vi "scan nufern reply string.vi"(0 "Input String":string, 2 "Manual":bool, 5 "error in (no error)":errorcluster={"status"=FALSE, "code"=0, "source"="No Error."}) -> (6 "Laser is in High Power Mode":bool, 8 "Status Cluster":T2, 9 "HPE Photodiode Reading":u32 format="0x%08x", 10 "Fault Cluster":T1, 11 "Back-Reflection Reading":u32 format="0x%08x", 13 "Return Code Cluster":T7 {"Current RS-485 \nAddress" format="0x%02x"; "Desired RS-485 \nAddress" format="0x%02x"; "Set Power Mode Return Code" format="0x%02x"; "Clear Faults Return Code" format="0x%02x"; "Return Code Description" items=["Accepted/No Error", "Incorrect Message Format", "Incorrect Message Length", "CRC Error", "Unrecognized Command", "Argument Out of Range", "Argument Parse Error", "Operation Not Permitted", "Operation Failed"]; "Get RS-485 Address \nReturn Code" format="0x%02x"; "Set RS-485 Address \nReturn Code" format="0x%02x"; "Set Power Mode Return Code" format="0x%02x"; "Clear Faults Return Code" format="0x%02x"; "Extended Status Return Code" format="0x%02x"}, 14 "New value is outside \nof the inclusive range of 1-99%":bool, 15 "New Value Could not be parsed":bool, 16 "Fault Status Cluster":T5, 17 "Extended Status Cluster":T4 {"Temperature Array" format="0x%02x"; "Back-Reflection" format="0x%08x"; "HPE Threshold" format="0x%08x"; "HPE Monitor" format="0x%08x"; "Stage 2 Output Monitor" format="0x%08x"; "Stage 1 Input Monitor" format="0x%08x"; "Stage 2 Current" format="0x%08x"; "Stage 1 Current" format="0x%08x"; "Extended Status Return Code" format="0x%02x"}, 18 "Unit Status Cluster":T6={"laser serial number"=0, "Firmware Part Number"=0, "Firmware Version Major"=1, "Firmware Version Minor"=1, "Firmware Version Bugfix"=1, "Gateware Part Number"=0, "Gateware Version Minor"=1, "Gateware Version Major"=1, "Gateware Version Bugfix"=1, "Valid Readings"=FALSE} {"Gateware Version Bugfix" format="0x%02x"; "Gateware Version Major" format="0x%02x"; "Gateware Version Minor" format="0x%02x"; "Gateware Part Number" format="0x%04x"; "Firmware Version Bugfix" format="0x%02x"; "Firmware Version Minor" format="0x%02x"; "Firmware Version Major" format="0x%02x"; "Firmware Part Number" format="0x%04x"}, 19 "error out":errorcluster)   [LabVIEW 2016]
uses:
  sniper current tests/Return Code Cluster.ctl
  2 digit hex indicator.ctl
  sniper current tests/Unit Status Cluster Control 1.ctl
  sniper current tests/Status  Cluster.ctl
  sniper current tests/Fault Cluster.ctl
panel:
  out "Logistics":u16(ring)=65 items=["Set RS-485 Address"=65, "Get RS-485 Address"=66]
  out "Common Operation":u16(ring) items=["undetermined", "Get Unit Information", "Emission On", "Emission Off", "Get Basic Status", "Get Core Status", "Get Extended Status", "Clear Faults", "Set Power Mode", ""]
  out "remaining string":string
  out "return code":u32 format="0x%02x"
  in  "String":string
  out "hexadecimal string out":string
  out "CRC Out":i32 format="0x%x"
  out "CRC Valid":bool
  out "Calculated CRC":i32 format="0x%x"
  out "Response string":string
  out "Address  String Out":string
  out "ID word":u32 format="0x%02x"
  out "Address Integer":u32 format="0x%02x"
  out "after address":string
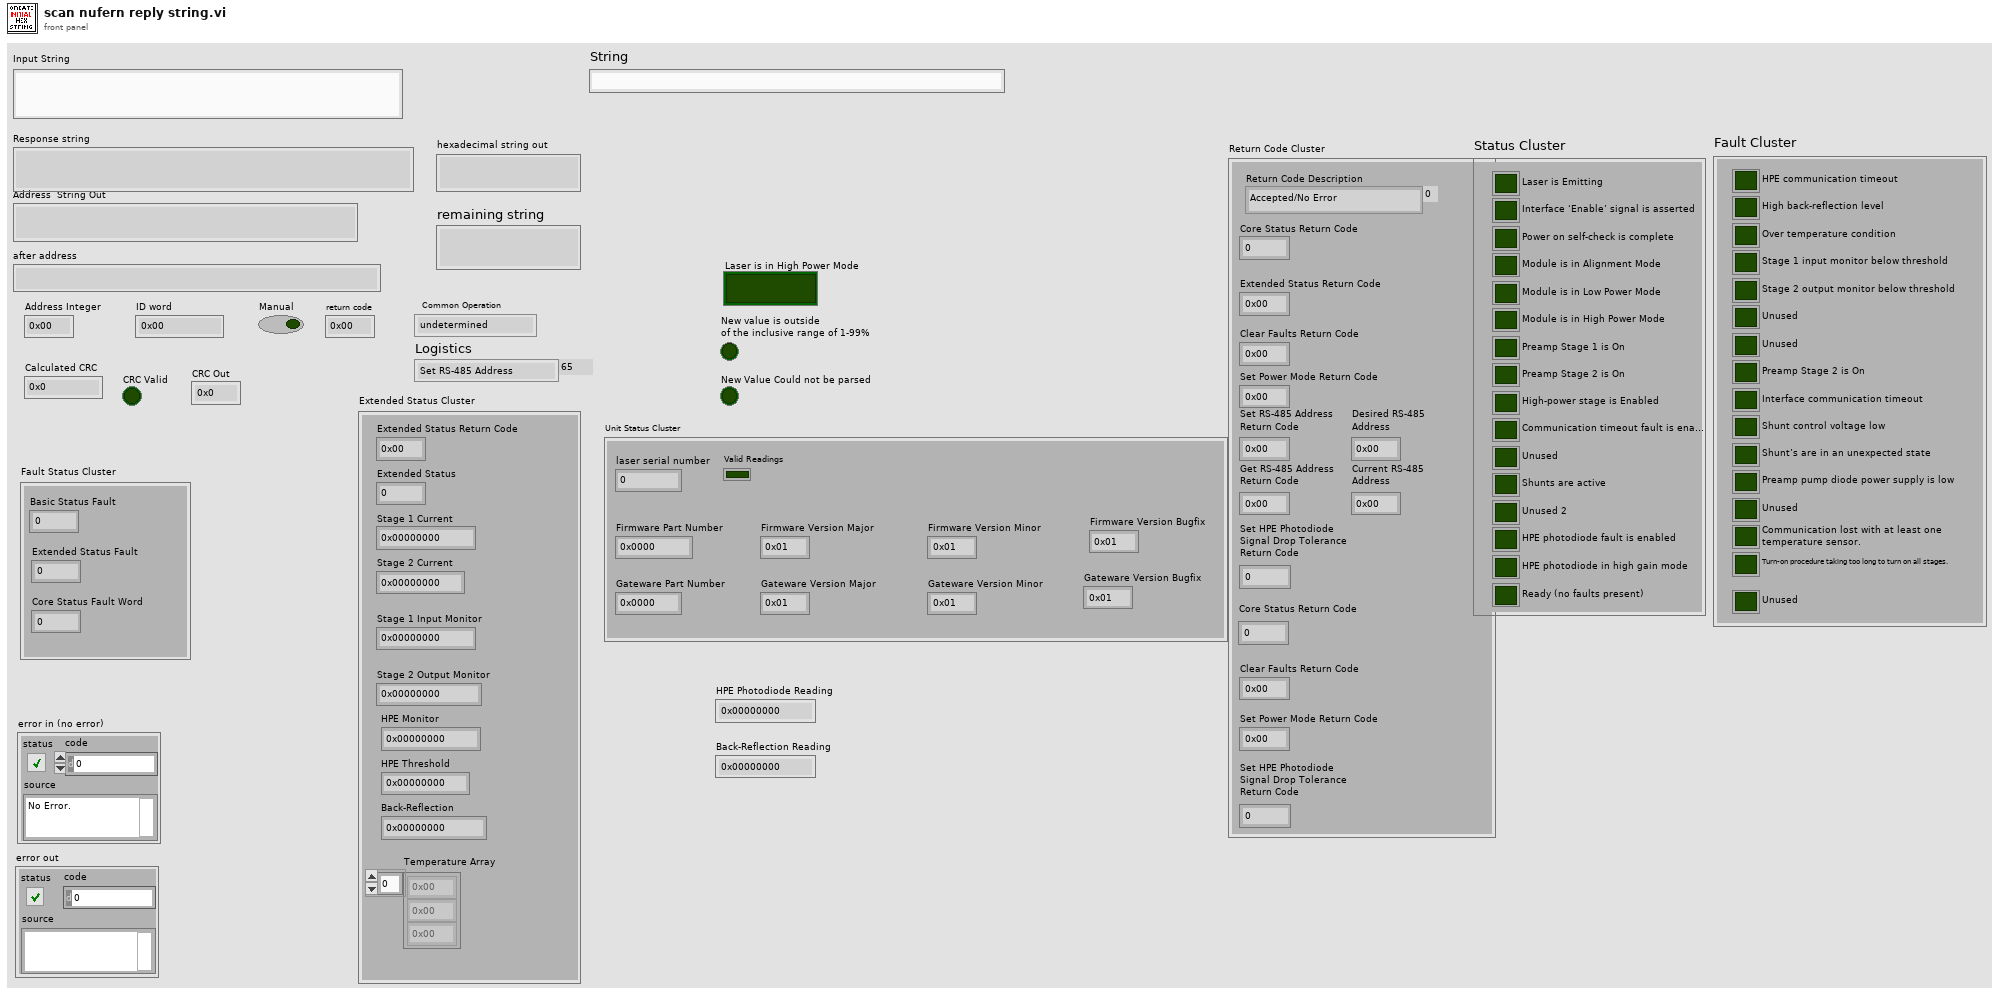
[diagram p1: front panel]
types:
  T1 = typedef "Fault Cluster.ctl" = cluster{"HPE communication timeout":bool, "High back-reflection level":bool, "Over temperature condition":bool, "Stage 1 input monitor below threshold":bool, "Stage 2 output monitor below threshold":bool, "Unused":bool, "Unused":bool, "Preamp Stage 2 is On":bool, "Interface communication timeout":bool, "Shunt control voltage low":bool, "Shunt’s are in an unexpected state":bool, "Preamp pump diode power supply is low":bool, "Unused":bool, "Communication lost with at least one\ntemperature sensor.":bool, "Turn-on procedure taking too long to turn on all stages.":bool, "Unused":bool}
  T2 = typedef "Status  Cluster.ctl" = cluster{"Laser is Emitting":bool, "Interface ‘Enable’ signal is asserted":bool, "Power on self-check is complete":bool, "Module is in Alignment Mode":bool, "Module is in Low Power Mode":bool, "Module is in High Power Mode":bool, "Preamp Stage 1 is On":bool, "Preamp Stage 2 is On":bool, "High-power stage is Enabled":bool, "Communication timeout fault is enabled":bool, "Unused":bool, "Shunts are active":bool, "Unused 2":bool, "HPE photodiode fault is enabled":bool, "HPE photodiode in high gain mode":bool, "Ready (no faults present)":bool}
  T3 = typedef "2 digit hex indicator.ctl" = i32
  T4 = cluster{"Extended Status Return Code":T3, "Extended Status ":u32, "Stage 1 Current":u32, "Stage 2 Current":u32, "Stage 1 Input Monitor":u32, "Stage 2 Output Monitor":u32, "HPE Monitor":u32, "HPE Threshold":u32, "Back-Reflection":u32, "Temperature Array":T3[]}
  T5 = cluster{"Basic Status Fault":u32, "Core Status Fault Word":u32, "Extended Status Fault":u32}
  T6 = typedef "Unit Status Cluster Control 1.ctl" = cluster{"laser serial number":u32, "Firmware Part Number":u32, "Firmware Version Major":T3, "Firmware Version Minor":T3, "Firmware Version Bugfix":T3, "Gateware Part Number":u32, "Gateware Version Minor":T3, "Gateware Version Major":T3, "Gateware Version Bugfix":T3, "Valid Readings":bool}
  T7 = typedef "Return Code Cluster.ctl" = cluster{"Core Status Return Code":u32, "Extended Status Return Code":T3, "Clear Faults Return Code":T3, "Set Power Mode Return Code":T3, "Set RS-485 Address \nReturn Code":T3, "Get RS-485 Address \nReturn Code":T3, "Set HPE Photodiode \nSignal Drop Tolerance \nReturn Code":u32, "Return Code Description":u16, "Core Status Return Code":u32, "Clear Faults Return Code":T3, "Set Power Mode Return Code ":T3, "Desired RS-485 \nAddress ":T3, "Current RS-485 \nAddress ":T3, "Set HPE Photodiode \nSignal Drop Tolerance \nReturn Code ":u32}
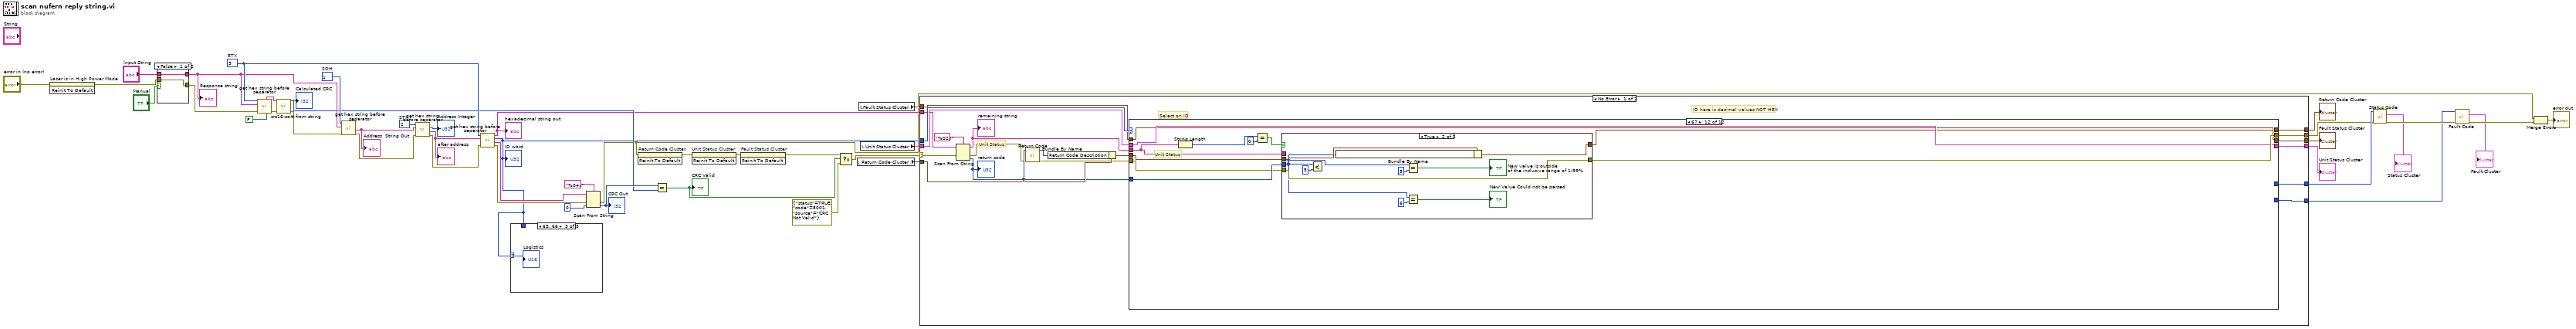
[diagram p0: block diagram]
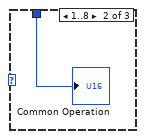
[diagram p3: hidden frame]
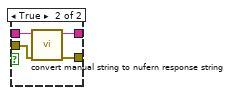
[diagram p4: hidden frame]
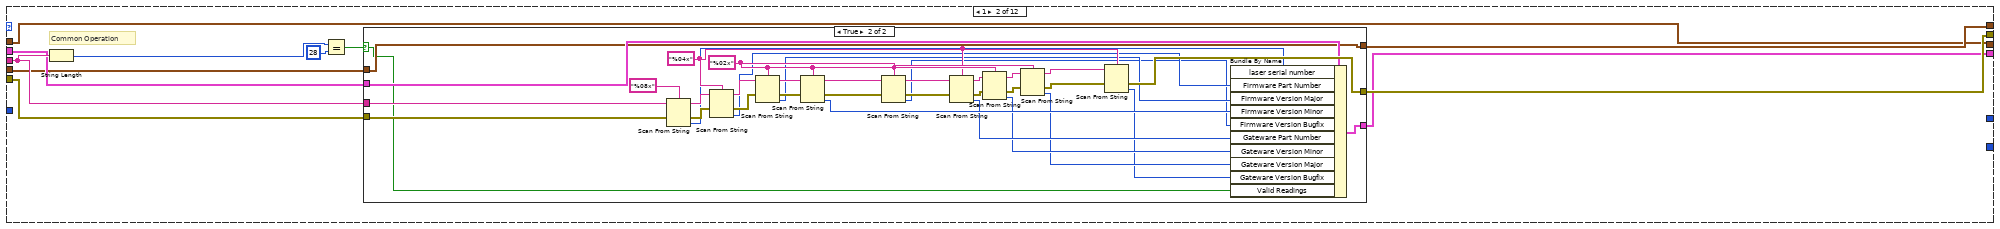
[diagram p6: hidden frame]
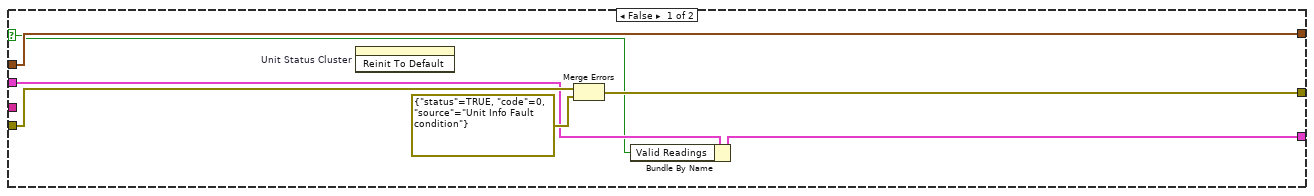
[diagram p7: hidden frame]
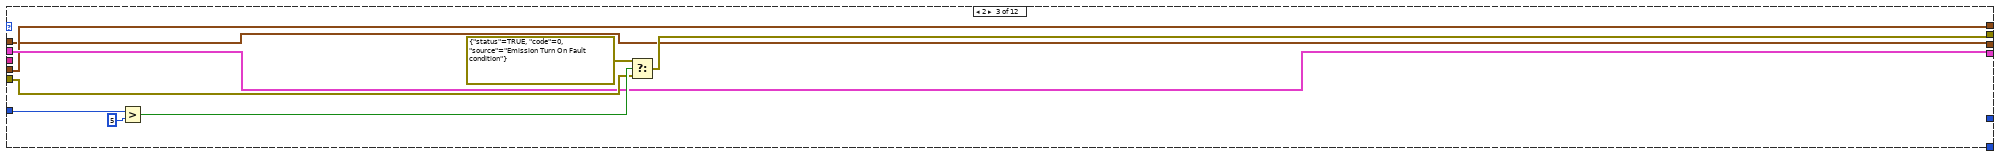
[diagram p8: hidden frame]
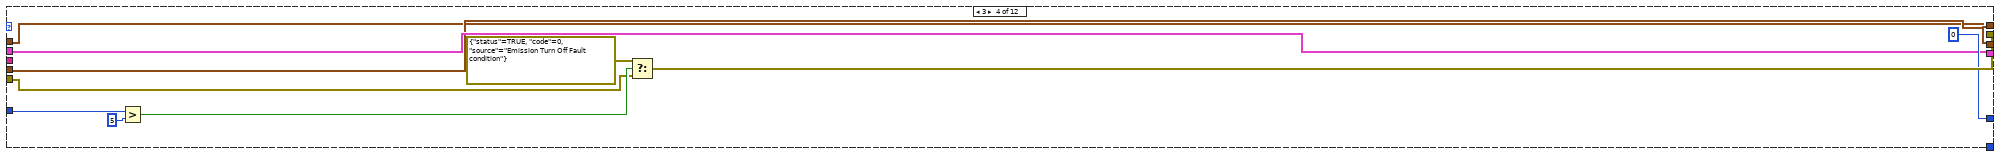
[diagram p9: hidden frame]
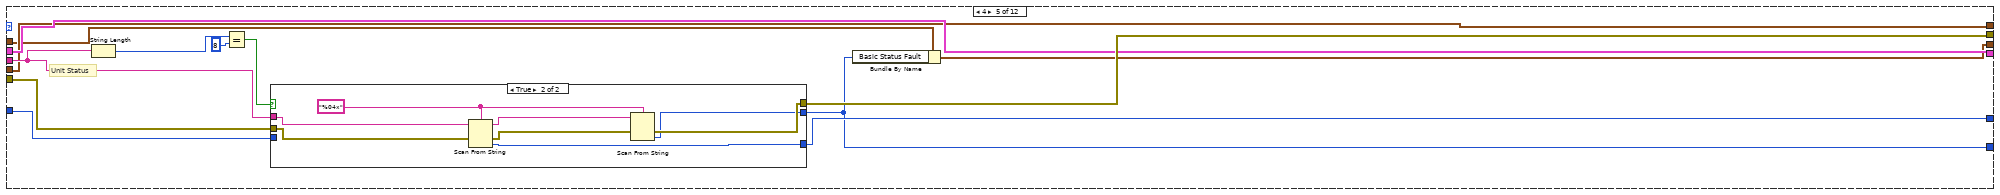
[diagram p10: hidden frame]
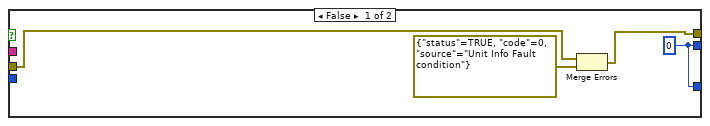
[diagram p11: hidden frame]
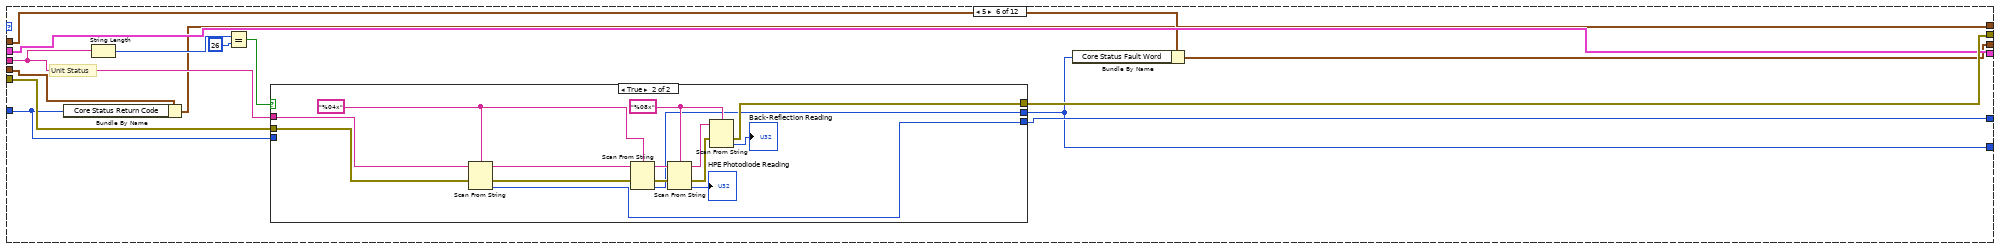
[diagram p12: hidden frame]
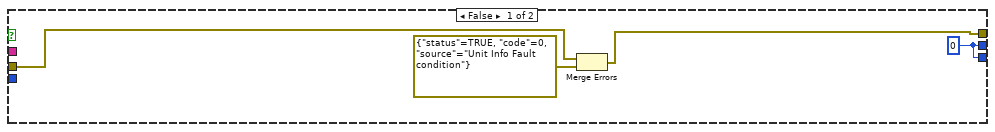
[diagram p13: hidden frame]
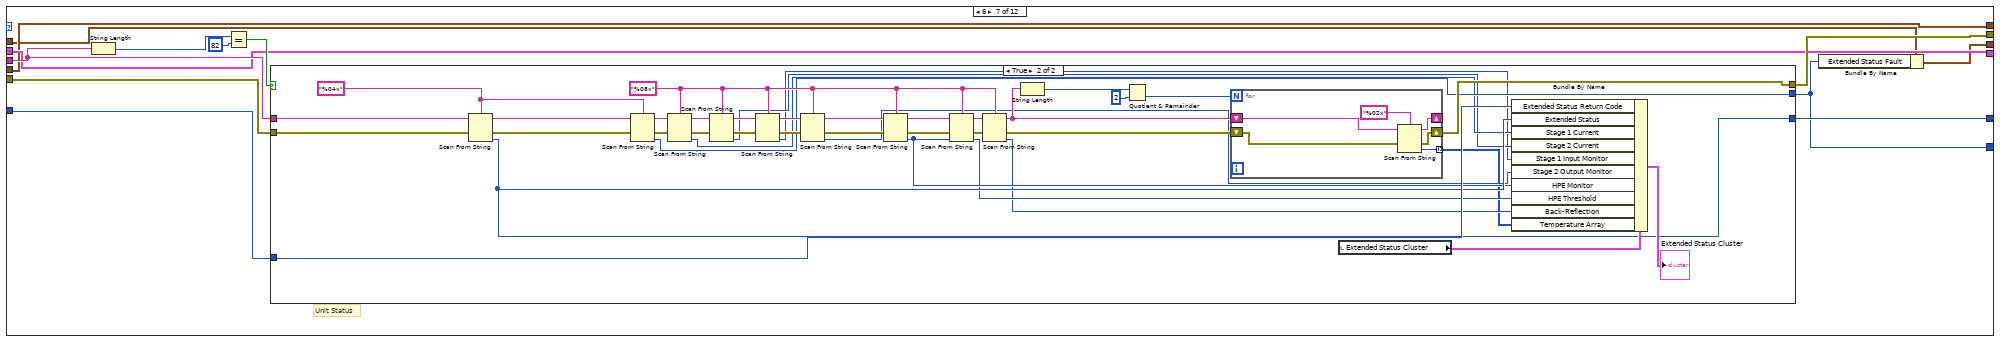
[diagram p14: hidden frame]
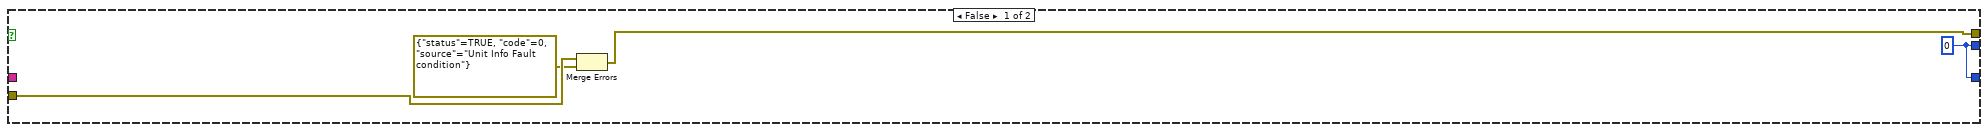
[diagram p15: hidden frame]
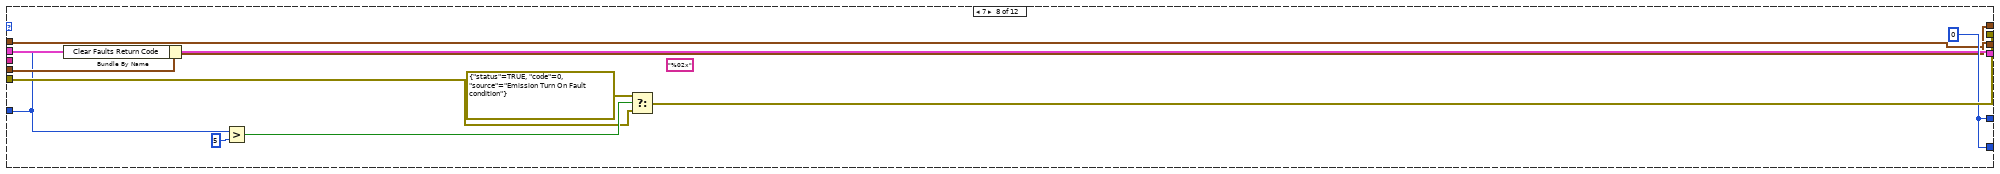
[diagram p16: hidden frame]
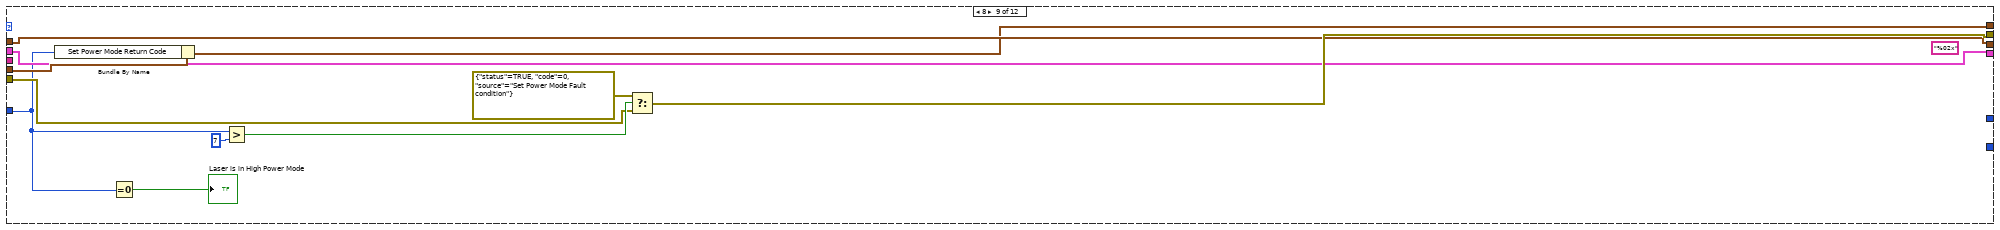
[diagram p17: hidden frame]
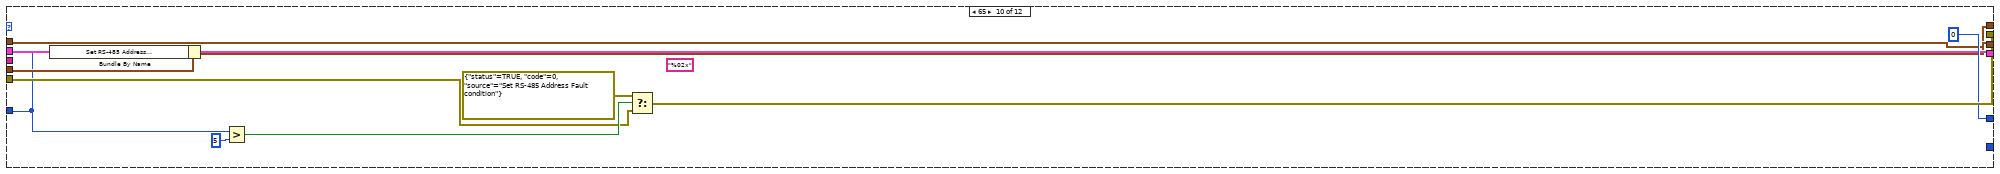
[diagram p18: hidden frame]
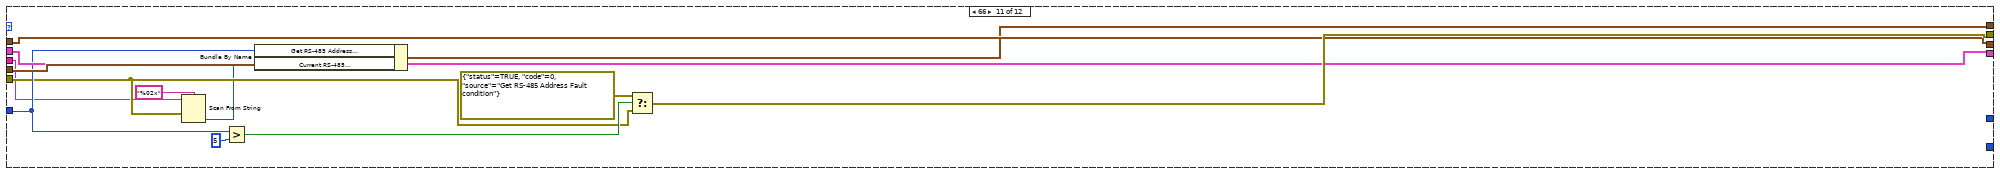
[diagram p19: hidden frame]
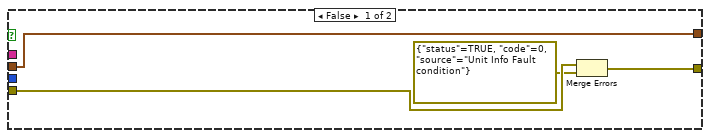
[diagram p20: hidden frame]
diagram:
  w41 = 3  # ETX
  w47 = 2  # STX
  w45 = 1  # SOH
  n1 = invoke on="Laser is in High Power Mode" class="Bool (strict)" method="Reinit To Default"(error in="error in (no error)") -> (error out=w11:errorcluster)  [unwired: 2 in, 2 out]
  n2 = case shown="False" "Manual" {
    tunnel: "Input String" -> [w48 w53]
    tunnel: w11 -> [w49 w52]
    tunnel: [w49 w51] -> w40
    tunnel: [w48 w50] -> w39
    frame False {
    }
    frame True {
      n3 = call "convert manual string to nufern response string.vi"("error in (no error)"=w52, "Manual String"=w53) -> ("error out"=w51:errorcluster, "result string"=w50:string)  [unwired: 8 in]
    }
  }
  "Response string" <- w39
  n4 = call "get hex string before separator.vi"("Convert to hex?"=FALSE, "error in (no error)"=w40, "String In"=w39, "Separator In"=w41) -> ("error out"=w38:errorcluster, "String Before and Separator"=w37:string)  [unwired: 3 in, 3 out]
  n5 = call "crc16-ccitt from string.vi"("error in (no error)"=w38, "String"=w37) -> ("error out"=w36:errorcluster, "CRC Out"=w29:i32)  [unwired: 8 in]
  "Calculated CRC" <- w29
  n6 = call "get hex string before separator.vi"("error in (no error)"=w36, "String In"=w39, "Separator In"=w45) -> ("error out"=w44:errorcluster, "after match out"=w43:string)  [unwired: 4 in, 3 out]
  "Address  String Out" <- w43
  n7 = call "get hex string before separator.vi"("error in (no error)"=w44, "String In"=w43, "Separator In"=w47) -> ("error out"=w9:errorcluster, "after match out"=w28:string, "hexadecimal 1 out"=→"Address Integer":u32)  [unwired: 4 in, 2 out]
  "after address" <- w28
  n8 = call "get hex string before separator.vi"("error in (no error)"=w9, "String In"=w28, "Separator In"=w41) -> ("error out"=w32:errorcluster, "after match out"=w34:string, "hexadecimal 1 out"=w1:u32, "hexadecimal string out"=w10:string)  [unwired: 4 in, 1 out]
  "ID word" <- w1
  "hexadecimal string out" <- w10
  n9 = case shown="65, 66" w1 {
    selector: w1 -> [_ _ w55]
    tunnel: w1 -> [_ w54 _]
    frame 0, Default {
    }
    frame 1..8 {
      "Common Operation" <- w54
    }
    frame 65, 66 {
      "Logistics" <- w55
    }
  }
  n10 = Scan From String(format string="%04x", input string=w34, error in=w32, default 1=0 ("default value 1")) -> (error out=w4:errorcluster, output 1=w30:i32)  [unwired: 1 in, 2 out]
  "CRC Out" <- w30
  n11 = invoke on="Return Code Cluster" class="Clust (strict)" method="Reinit To Default"(error in=w4) -> (error out=w14:errorcluster)  [unwired: 2 in, 2 out]
  n12 = Equal?(x=w30, y=w29) -> (x = y?=w7:bool)
  "CRC Valid" <- w7
  n13 = invoke on="Unit Status Cluster" class="Clust (strict)" method="Reinit To Default"(error in=w14) -> (error out=w13:errorcluster)  [unwired: 2 in, 2 out]
  n14 = invoke on="Fault Status Cluster" class="Clust (strict)" method="Reinit To Default"(error in=w13) -> (error out=w6:errorcluster)  [unwired: 2 in, 2 out]
  n15 = Select(t=w6, s=w7, f=errorcluster {"status"=TRUE, "code"=8001, "source"="CRC Not Valid"}) -> (s? t:f=w8:errorcluster)
  n16 = local read "Return Code Cluster"() -> (w19:T7)
  n17 = local read "Fault Status Cluster"() -> (w16:T5)
  n18 = local read "Unit Status Cluster"() -> (w17:T6)
  n19 = case shown="No Error" w8 {
    selector: w8 -> [w70 w345]
    tunnel: w1 -> [w74 _]
    tunnel: w10 -> [w71 _]
    tunnel: [w73 w345] -> w26
    tunnel: [w68 u32 0] -> w27
    tunnel: [w67 _] -> w22
    tunnel: [w66 w343] -> w20
    tunnel: w19 -> [w65 w343]
    tunnel: [w63 w342] -> w18
    tunnel: w17 -> [w62 w342]
    tunnel: w16 -> [w61 w341]
    tunnel: [w60 w341] -> w15
    frame No Error {
      # "ID here is decimal values NOT HEX"
      # "Select on ID"
      # "Unit Status"
      n20 = Scan From String(format string="%02x", input string=w71, error in=w70) -> (remaining string=w69:string, error out=w58:errorcluster, output 1=w59:u32)  [unwired: 2 in, 1 out]
      "return code" <- w59
      "remaining string" <- w69
      n21 = call "Return Code.vi"("error in (no error)"=w58, "Return Code"=w59) -> ("error out"=w57:errorcluster, "Return Code Description"=w56:u16)  [unwired: 8 in]
      n22 = Bundle By Name(cluster=w65, "Return Code Description"=w56) -> (w64:T7)
      n23 = case shown="67" w74 {
        tunnel: w69 -> [_ w85 _ _ w162 w188 w220 _ _ _ w305 w326]
        tunnel: [w78 w89 w137 w147 w163 w189 w221 w278 w289 w300 w313 w327] -> w73
        tunnel: w57 -> [w78 w84 w135 w145 w157 w184 w215 w277 w287 w299 w307 w321]
        tunnel: w59 -> [_ _ w136 w146 w158 w176 w216 w271 w282 w293 w308 w322]
        tunnel: [_ _ _ u32 0 w156 w183 w214 w276 _ u32 0 _ _] -> w68
        tunnel: [_ _ _ _ w151 w178 w209 w276 _ _ _ _] -> w67
        tunnel: [w77 w80 w133 w142 w154 w177 w212 w272 w283 w294 w309 w317] -> w66
        tunnel: w64 -> [w77 w81 w133 w142 w154 w181 w212 w275 w286 w297 w312 w318]
        tunnel: [w76 w82 w134 w143 w155 w182 w213 w274 w285 w296 w311 w320] -> w63
        tunnel: w62 -> [w76 w83 w134 w143 w155 w182 w213 w274 w285 w296 w311 w320]
        tunnel: w61 -> [w75 w79 w132 w141 w153 w180 w211 w273 w284 w295 w310 w319]
        tunnel: [w75 w79 w132 w141 w152 w179 w210 w273 w284 w295 w310 w319] -> w60
        frame 0, Default {
        }
        frame 1 {
          # "Common Operation"
          n24 = String Length(string=w85) -> (length=w88:i32)
          n25 = Equal?(x=w88, y=28) -> (x = y?=w87:bool)
          n26 = case shown="True" w87 {
            selector: w87 -> [w90 w97]
            tunnel: w84 -> [w96 w110]
            tunnel: [w95 w112] -> w89
            tunnel: w85 -> [_ w111]
            tunnel: w83 -> [w93 w109]
            tunnel: [w91 w107] -> w82
            tunnel: w81 -> [w92 w108]
            tunnel: [w92 w108] -> w80
            frame False {
              n27 = invoke on="Unit Status Cluster" class="Clust (strict)" method="Reinit To Default"() -> ()  [unwired: 3 in, 3 out]
              n28 = Merge Errors(w96, errorcluster {"status"=TRUE, "code"=0, "source"="Unit Info Fault condition"} ("t")) -> (w95:errorcluster)
              n29 = Bundle By Name(cluster=w93, "Valid Readings"=w90) -> (w91:T6)
            }
            frame True {
              w116 = "%02x" ("format string")
              w115 = "%04x" ("format string")
              n30 = Scan From String(format string="%08x", input string=w111, error in=w110) -> (remaining string=w129:string, error out=w130:errorcluster, output 1=w106:u32)  [unwired: 2 in, 1 out]
              n31 = Scan From String(format string=w115, input string=w129, error in=w130) -> (remaining string=w128:string, error out=w127:errorcluster, output 1=w105:u32)  [unwired: 2 in, 1 out]
              n32 = Scan From String(format string=w116, input string=w128, error in=w127) -> (remaining string=w126:string, error out=w125:errorcluster, output 1=w104:u32)  [unwired: 2 in, 1 out]
              n33 = Scan From String(format string=w116, input string=w126, error in=w125) -> (remaining string=w123:string, error out=w124:errorcluster, output 1=w103:u32)  [unwired: 2 in, 1 out]
              n34 = Scan From String(format string=w116, input string=w123, error in=w124) -> (remaining string=w121:string, error out=w122:errorcluster, output 1=w102:u32)  [unwired: 2 in, 1 out]
              n35 = Scan From String(format string=w115, input string=w121, error in=w122) -> (remaining string=w118:string, error out=w120:errorcluster, output 1=w101:u32)  [unwired: 2 in, 1 out]
              n36 = Scan From String(format string=w116, input string=w118, error in=w120) -> (remaining string=w117:string, error out=w119:errorcluster, output 1=w100:u32)  [unwired: 2 in, 1 out]
              n37 = Scan From String(format string=w116, input string=w117, error in=w119) -> (remaining string=w114:string, error out=w113:errorcluster, output 1=w99:u32)  [unwired: 2 in, 1 out]
              n38 = Scan From String(format string=w115, input string=w114, error in=w113) -> (error out=w112:errorcluster, output 1=w98:u32)  [unwired: 2 in, 2 out]
              n39 = Bundle By Name(cluster=w109, "laser serial number"=w106, "Firmware Part Number"=w105, "Firmware Version Major"=w104, "Firmware Version Minor"=w103, "Firmware Version Bugfix"=w102, "Gateware Part Number"=w101, "Gateware Version Minor"=w100, "Gateware Version Major"=w99, "Gateware Version Bugfix"=w98, "Valid Readings"=w97) -> (w107:T6)
            }
          }
        }
        frame 2 {
          n40 = Greater?(x=w136, y=T3 5) -> (0:w139:bool)
          n41 = Select(t=errorcluster {"status"=TRUE, "code"=0, "source"="Emission Turn On Fault condition"}, s=w139, f=w135) -> (s? t:f=w137:errorcluster)
        }
        frame 3 {
          n42 = Greater?(x=w146, y=T3 5) -> (0:w149:bool)
          n43 = Select(t=errorcluster {"status"=TRUE, "code"=0, "source"="Emission Turn Off Fault condition"}, s=w149, f=w145) -> (s? t:f=w147:errorcluster)
        }
        frame 4 {
          # "Unit Status"
          n44 = String Length(string=w162) -> (length=w161:i32)
          n45 = Equal?(x=w161, y=8) -> (x = y?=w160:bool)
          n46 = case shown="True" w160 {
            tunnel: w157 -> [w167 w170]
            tunnel: [w166 w173] -> w163
            tunnel: w162 -> [_ w171]
            tunnel: w158 -> [_ _]
            tunnel: [w164 w169] -> w156
            tunnel: [w164 w168] -> w151
            frame False {
              w164 = u32 0
              n47 = Merge Errors(w167, errorcluster {"status"=TRUE, "code"=0, "source"="Unit Info Fault condition"} ("t")) -> (w166:errorcluster)
            }
            frame True {
              w172 = "%04x" ("format string")
              n48 = Scan From String(format string=w172, input string=w171, error in=w170) -> (remaining string=w175:string, error out=w174:errorcluster, output 1=w169:u32)  [unwired: 2 in, 1 out]
              n49 = Scan From String(format string=w172, input string=w175, error in=w174) -> (error out=w173:errorcluster, output 1=w168:u32)  [unwired: 2 in, 2 out]
            }
          }
          n50 = Bundle By Name(cluster=w153, "Basic Status Fault"=w151) -> (w152:T5)
        }
        frame 5 {
          # "Unit Status"
          n51 = Bundle By Name(cluster=w181, "Core Status Return Code"=w176) -> (w177:T7)
          n52 = String Length(string=w188) -> (length=w187:i32)
          n53 = Equal?(x=w187, y=26) -> (x = y?=w186:bool)
          n54 = case shown="True" w186 {
            tunnel: w184 -> [w193 w197]
            tunnel: [w192 w200] -> w189
            tunnel: w188 -> [_ w196]
            tunnel: w176 -> [_ _]
            tunnel: [w190 w195] -> w178
            tunnel: [w190 w194] -> w183
            frame False {
              w190 = u32 0
              n55 = Merge Errors(w193, errorcluster {"status"=TRUE, "code"=0, "source"="Unit Info Fault condition"} ("t")) -> (w192:errorcluster)
            }
            frame True {
              w199 = "%08x" ("format string")
              w206 = "%04x" ("format string")
              n56 = Scan From String(format string=w206, input string=w196, error in=w197) -> (remaining string=w208:string, error out=w207:errorcluster, output 1=w194:u32)  [unwired: 2 in, 1 out]
              n57 = Scan From String(format string=w206, input string=w208, error in=w207) -> (remaining string=w205:string, error out=w204:errorcluster, output 1=w195:u32)  [unwired: 2 in, 1 out]
              n58 = Scan From String(format string=w199, input string=w205, error in=w204) -> (remaining string=w201:string, error out=w202:errorcluster, output 1=→"HPE Photodiode Reading":u32)  [unwired: 2 in, 1 out]
              n59 = Scan From String(format string=w199, input string=w201, error in=w202) -> (error out=w200:errorcluster, output 1=→"Back-Reflection Reading":u32)  [unwired: 2 in, 2 out]
            }
          }
          n60 = Bundle By Name(cluster=w180, "Core Status Fault Word"=w178) -> (w179:T5)
        }
        frame 6 {
          # "Unit Status"
          n61 = String Length(string=w220) -> (length=w219:i32)
          n62 = Equal?(x=w219, y=82) -> (x = y?=w218:bool)
          n63 = case shown="True" w218 {
            tunnel: w215 -> [w225 w244]
            tunnel: [w224 w245] -> w221
            tunnel: w220 -> [_ w243]
            tunnel: w216 -> [_ w235]
            tunnel: [w222 w234] -> w214
            tunnel: [w222 w238] -> w209
            frame False {
              w222 = 0
              n64 = Merge Errors(w225, errorcluster {"status"=TRUE, "code"=0, "source"="Unit Info Fault condition"} ("t")) -> (w224:errorcluster)
            }
            frame True {
              w248 = "%08x" ("format string")
              w262 = "%04x" ("format string")
              n65 = Scan From String(format string=w262, input string=w243, error in=w244) -> (remaining string=w264:string, error out=w263:errorcluster, output 1=w234:u32)  [unwired: 2 in, 1 out]
              n66 = Scan From String(format string=w262, input string=w264, error in=w263) -> (remaining string=w261:string, error out=w260:errorcluster, output 1=w238:u32)  [unwired: 2 in, 1 out]
              n67 = Scan From String(format string=w248, input string=w261, error in=w260) -> (remaining string=w258:string, error out=w259:errorcluster, output 1=w233:u32)  [unwired: 2 in, 1 out]
              n68 = Scan From String(format string=w248, input string=w258, error in=w259) -> (remaining string=w256:string, error out=w254:errorcluster, output 1=w232:u32)  [unwired: 2 in, 1 out]
              n69 = Scan From String(format string=w248, input string=w256, error in=w254) -> (remaining string=w255:string, error out=w257:errorcluster, output 1=w231:u32)  [unwired: 2 in, 1 out]
              n70 = Scan From String(format string=w248, input string=w255, error in=w257) -> (remaining string=w247:string, error out=w253:errorcluster, output 1=w230:u32)  [unwired: 2 in, 1 out]
              n71 = Scan From String(format string=w248, input string=w247, error in=w253) -> (remaining string=w250:string, error out=w252:errorcluster, output 1=w229:u32)  [unwired: 2 in, 1 out]
              n72 = Scan From String(format string=w248, input string=w250, error in=w252, default 1=w229) -> (remaining string=w249:string, error out=w251:errorcluster, output 1=w228:u32)  [unwired: 1 in, 1 out]
              n73 = Scan From String(format string=w248, input string=w249, error in=w251) -> (remaining string=w242:string, error out=w246:errorcluster, output 1=w227:u32)  [unwired: 2 in, 1 out]
              n74 = String Length(string=w242) -> (length=w240:i32)
              n75 = Quotient & Remainder(x=w240, y=2) -> (floor(x/y)=w241:i32)  [unwired: 1 out]
              n76 = for {
                N: w241 -> [_]
                shift-right: [w268] -> _
                shift-left: w242 -> [w269]
                shift-right: [w266] -> w245
                shift-left: w246 -> [w267]
                tunnel: [w265] -> w226 mode=indexing
                n77 = Scan From String(format string="%02x", input string=w269, error in=w267) -> (remaining string=w268:string, error out=w266:errorcluster, output 1=w265:u32)  [unwired: 2 in, 1 out]
              }
              n78 = local read "Extended Status Cluster"() -> (w237:T4)
              n79 = Bundle By Name(cluster=w237, "Extended Status Return Code"=w235, "Extended Status"=w234, "Stage 1 Current"=w233, "Stage 2 Current"=w232, "Stage 1 Input Monitor"=w231, "Stage 2 Output Monitor"=w230, "HPE Monitor"=w229, "HPE Threshold"=w228, "Back-Reflection"=w227, "Temperature Array"=w226) -> (→"Extended Status Cluster":T4)
            }
          }
          n80 = Bundle By Name(cluster=w211, "Extended Status Fault"=w209) -> (w210:T5)
        }
        frame 7 {
          w276 = u32 0
          (unwired) "%02x" ("format string")
          n81 = Bundle By Name(cluster=w275, "Clear Faults Return Code"=w271) -> (w272:T7)
          n82 = Greater?(x=w271, y=T3 5) -> (0:w280:bool)
          n83 = Select(t=errorcluster {"status"=TRUE, "code"=0, "source"="Emission Turn On Fault condition"}, s=w280, f=w277) -> (s? t:f=w278:errorcluster)
        }
        frame 8 {
          (unwired) "%02x" ("format string")
          n84 = Bundle By Name(cluster=w286, "Set Power Mode Return Code"=w282) -> (w283:T7)
          n85 = Equal To 0?(x=w282) -> (x = 0?=→"Laser is in High Power Mode":bool)
          n86 = Greater?(x=w282, y=T3 7) -> (0:w291:bool)
          n87 = Select(t=errorcluster {"status"=TRUE, "code"=0, "source"="Set Power Mode Fault condition"}, s=w291, f=w287) -> (s? t:f=w289:errorcluster)
        }
        frame 65 {
          (unwired) "%02x" ("format string")
          n88 = Bundle By Name(cluster=w297, "Set RS-485 Address \nReturn Code"=w293) -> (w294:T7)
          n89 = Greater?(x=w293, y=T3 5) -> (0:w302:bool)
          n90 = Select(t=errorcluster {"status"=TRUE, "code"=0, "source"="Set RS-485 Address Fault condition"}, s=w302, f=w299) -> (s? t:f=w300:errorcluster)
        }
        frame 66 {
          n91 = Scan From String(format string="%02x", input string=w305, error in=w307) -> (output 1=w304:u32)  [unwired: 2 in, 3 out]
          n92 = Greater?(x=w308, y=T3 5) -> (0:w315:bool)
          n93 = Bundle By Name(cluster=w312, "Get RS-485 Address \nReturn Code"=w308, "Current RS-485 \nAddress"=w304) -> (w309:T7)
          n94 = Select(t=errorcluster {"status"=TRUE, "code"=0, "source"="Get RS-485 Address Fault condition"}, s=w315, f=w307) -> (s? t:f=w313:errorcluster)
        }
        frame 67 {
          # "Unit Status"
          n95 = String Length(string=w326) -> (length=w325:i32)
          n96 = Equal?(x=w325, y=0) -> (x = y?=w324:bool)
          n97 = case shown="True" w324 {
            tunnel: w321 -> [w331 w335]
            tunnel: [w330 w335] -> w327
            tunnel: w326 -> [_ _]
            tunnel: w322 -> [_ w332]
            tunnel: w318 -> [w328 w334]
            tunnel: [w328 w333] -> w317
            frame False {
              n98 = Merge Errors(w331, errorcluster {"status"=TRUE, "code"=0, "source"="Unit Info Fault condition"} ("t")) -> (w330:errorcluster)
            }
            frame True {
              n99 = Less?(x=w332, y=u32 5) -> ()  [unwired: 1 out]
              n100 = Bundle By Name(cluster=w334, "Set HPE Photodiode \nSignal Drop Tolerance \nReturn Code"=w332) -> (w333:T7)
              n101 = Equal?(x=w332, y=u32 5) -> (x = y?=→"New value is outside \nof the inclusive range of 1-99%":bool)
              n102 = Equal?(x=w332, y=u32 6) -> (x = y?=→"New Value Could not be parsed":bool)
            }
          }
        }
      }
    }
    frame Error {
    }
  }
  "Return Code Cluster" <- w20
  "Unit Status Cluster" <- w18
  "Fault Status Cluster" <- w15
  n103 = call "Status Code.vi"("error in (no error)"=w26, "Status Code"=w27) -> ("error out"=w24:errorcluster, "Status Cluster"=→"Status Cluster":T2)  [unwired: 8 in]
  n104 = call "Fault Code.vi"("error in (no error)"=w24, "Fault Code"=w22) -> ("error out"=w23:errorcluster, "Fault Cluster"=→"Fault Cluster":T1)  [unwired: 8 in]
  n105 = Merge Errors(w4, w23) -> (→"error out":errorcluster)
